vi "NI-DP__GetEmptyMessage.vi"() -> (3 "NI-DP__EmptyMessage":T1 {"Command" items=["0x01: Get Type & Hostname"=1, "0x03: Set IP 1"=3, "0x04: Set IP 2"=4, "0x08: Acknowledge"=8, "0x0A: Reboot"=10, "0x20: ???"=32, "0x21: ???"=33, "0xF2: System State"=242, "0xF4: System Details"=244]})   [LabVIEW 2014, in "hse-network.lvlib"]
doc: "____\nHAMPEL SOFTWARE ENGINEERING v0.7.0 (2018-07-16 18:12)"
uses:
  hse-network.lvlib
  NI-DP__MessageStructure.ctl
  NI-DP__Commands.ctl
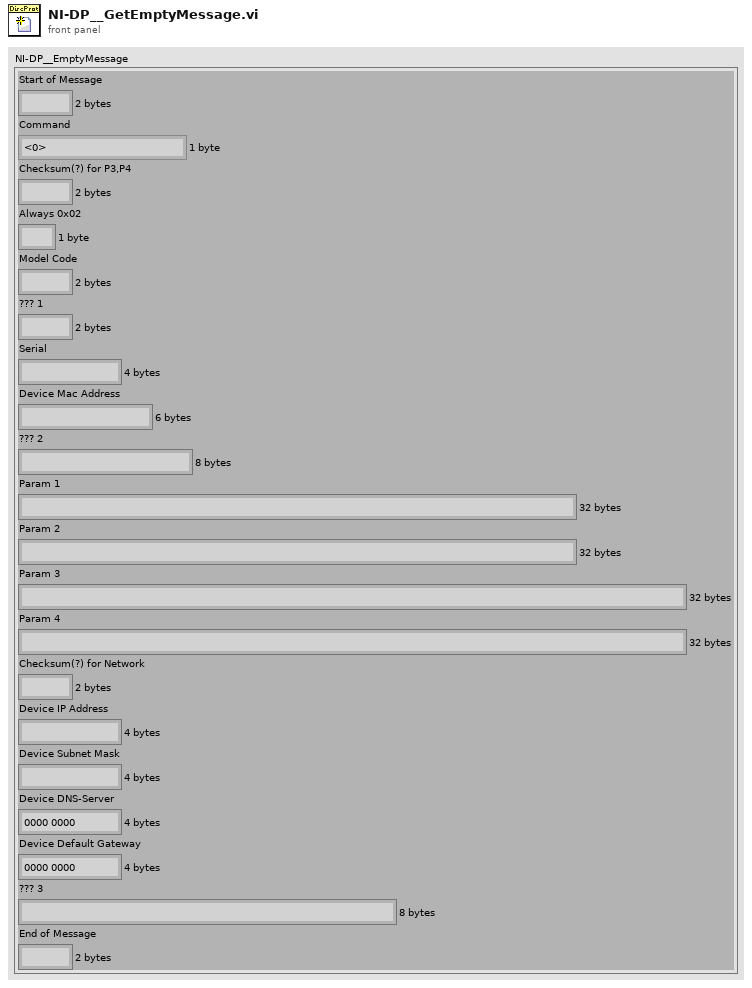
[diagram p1: front panel]
types:
  T1 = typedef "hse-network.lvlib/NI-DP__MessageStructure.ctl" = cluster{"Start of Message":string, "Command":T2, "Checksum(?) for P3,P4":string, "Always 0x02":string, "Model Code":string, "??? 1":string, "Serial":string, "Device Mac Address":string, "??? 2":string, "Param 1":string, "Param 2":string, "Param 3":string, "Param 4":string, "Checksum(?) for Network":string, "Device IP Address":string, "Device Subnet Mask":string, "Device DNS-Server":string, "Device Default Gateway":string, "??? 3":string, "End of Message":string}
  T2 = typedef "hse-network.lvlib/NI-DP__Commands.ctl" = u8
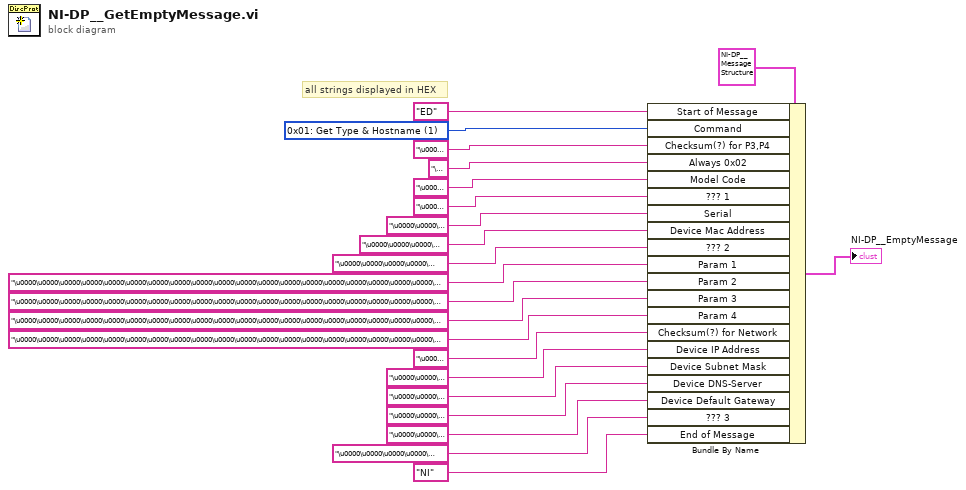
[diagram p0: block diagram]
diagram:
  w20 = T2 1 items=["0x01: Get Type & Hostname"=1, "0x03: Set IP 1"=3, "0x04: Set IP 2"=4, "0x08: Acknowledge"=8, "0x0A: Reboot"=10, "0x20: ???"=32, "0x21: ???"=33, "0xF2: System State"=242, "0xF4: System Details"=244] ("Command")
  # "all strings displayed in HEX"
  n1 = Bundle By Name(cluster=T1 {"Start of Message"="", "Command"=0, "Checksum(?) for P3,P4"="", "Always 0x02"="", "Model Code"="", "??? 1"="", "Serial"="", "Device Mac Address"="", "??? 2"="", "Param 1"="", "Param 2"="", "Param 3"="", "Param 4"="", "Checksum(?) for Network"="", "Device IP Address"="", "Device Subnet Mask"="", "Device DNS-Server"="", "Device Default Gateway"="", "??? 3"="", "End of Message"=""} ("NI-DP__MessageStructure"), "Start of Message"="ED", "Command"=w20, "Checksum(?) for P3,P4"="\u0000\u0000", "Always 0x02"="\u0002", "Model Code"="\u0000\u0000", "??? 1"="\u0000\u0000", "Serial"="\u0000\u0000\u0000\u0000", "Device Mac Address"="\u0000\u0000\u0000\u0000\u0000\u0000", "??? 2"="\u0000\u0000\u0000\u0000\u0000\u0000\u0000\u0000", "Param 1"="\u0000\u0000\u0000\u0000\u0000\u0000\u0000\u0000\u0000\u0000\u0000\u0000\u0000\u0000\u0000\u0000\u0000\u0000\u0000\u0000\u0000\u0000\u0000\u0000\u0000\u0000\u0000\u0000\u0000\u0000\u0000\u0000" ("Param 3"), "Param 2"="\u0000\u0000\u0000\u0000\u0000\u0000\u0000\u0000\u0000\u0000\u0000\u0000\u0000\u0000\u0000\u0000\u0000\u0000\u0000\u0000\u0000\u0000\u0000\u0000\u0000\u0000\u0000\u0000\u0000\u0000\u0000\u0000" ("Param 4"), "Param 3"="\u0000\u0000\u0000\u0000\u0000\u0000\u0000\u0000\u0000\u0000\u0000\u0000\u0000\u0000\u0000\u0000\u0000\u0000\u0000\u0000\u0000\u0000\u0000\u0000\u0000\u0000\u0000\u0000\u0000\u0000\u0000\u0000", "Param 4"="\u0000\u0000\u0000\u0000\u0000\u0000\u0000\u0000\u0000\u0000\u0000\u0000\u0000\u0000\u0000\u0000\u0000\u0000\u0000\u0000\u0000\u0000\u0000\u0000\u0000\u0000\u0000\u0000\u0000\u0000\u0000\u0000", "Checksum(?) for Network"="\u0000\u0000" ("Checksum(?) for IP"), "Device IP Address"="\u0000\u0000\u0000\u0000", "Device Subnet Mask"="\u0000\u0000\u0000\u0000", "Device DNS-Server"="\u0000\u0000\u0000\u0000" ("Device IP Address"), "Device Default Gateway"="\u0000\u0000\u0000\u0000" ("Device Subnet Mask"), "??? 3"="\u0000\u0000\u0000\u0000\u0000\u0000\u0000\u0000", "End of Message"="NI") -> (→"NI-DP__EmptyMessage":T1)
